vi "find worksheet index from name.vi"(8 "error in (no error)":errorcluster, 10 "Worksheet Name in":string, 11 "Worksheet Names":string[](array[string])) -> (0 "error out":errorcluster, 3 "Select Worksheet Index":i32)   [LabVIEW 2016]
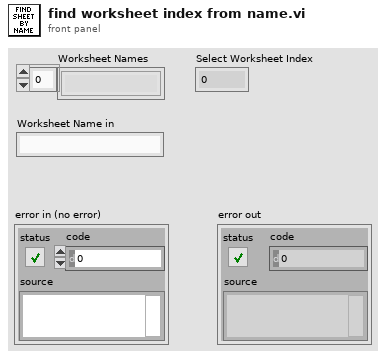
[diagram p1: front panel]
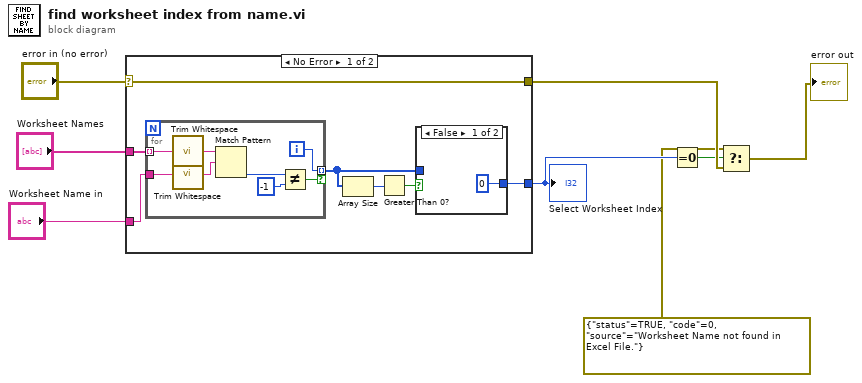
[diagram p0: block diagram]
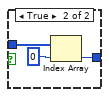
[diagram p2: hidden frame]
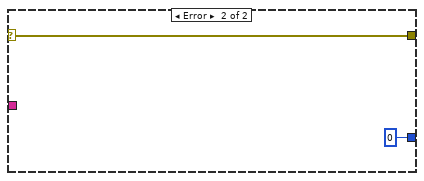
[diagram p3: hidden frame]
diagram:
  n1 = case shown="No Error" "error in (no error)" {
    selector: "error in (no error)" -> [w12 w28]
    tunnel: [w15 0] -> w2
    tunnel: "Worksheet Names" -> [w14 _]
    tunnel: "Worksheet Name in" -> [w13 _]
    tunnel: [w12 w28] -> w5
    frame No Error {
      n2 = for {
        tunnel: w14 -> [w27] mode=indexing
        tunnel: w13 -> [w26]
        tunnel: [w21] -> w11 mode=indexing if=w20
        i -> [w21]
        n3 = call <vilib>:"Trim Whitespace.vi"("string"=w27) -> ("trimmed string"=w25:string)  [unwired: 1 in]
        n4 = call <vilib>:"Trim Whitespace.vi"("string"=w26) -> ("trimmed string"=w24:string)  [unwired: 1 in]
        n5 = Match Pattern(string=w25, regular expression=w24) -> (offset past match=w23:i32)  [unwired: 1 in, 3 out]
        n6 = Not Equal?(x=w23, y=-1) -> (x != y?=w20:bool)
      }
      n7 = Array Size(array=w11) -> (size(s)=w10:i32)
      n8 = Greater Than 0?(x=w10) -> (x > 0?=w9:bool)
      n9 = case shown="False" w9 {
        tunnel: [0 w19] -> w15
        tunnel: w11 -> [_ w17]
        frame False {
        }
        frame True {
          n10 = Index Array(array=w17, index=0) -> (element=w19:i32)
        }
      }
    }
    frame Error {
    }
  }
  "Select Worksheet Index" <- w2
  n11 = Equal To 0?(x=w2) -> (x = 0?=w3:bool)
  n12 = Select(t=errorcluster {"status"=TRUE, "code"=0, "source"="Worksheet Name not found in Excel File."}, s=w3, f=w5) -> (s? t:f=→"error out":errorcluster)
